vi "WaitForBytes.vi"(8 "error in (no error)":errorcluster, 10 "timeout [s]":i32, 11 "VISA Refnum in":refnum<visa-resource-name>) -> (0 "error out":errorcluster, 2 "Bytes at Port":u32, 3 "VISA Refnum out":refnum<visa-resource-name>)   [LabVIEW 2016]
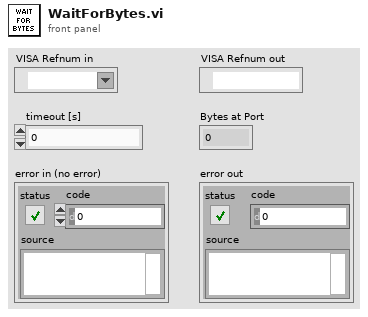
[diagram p1: front panel]
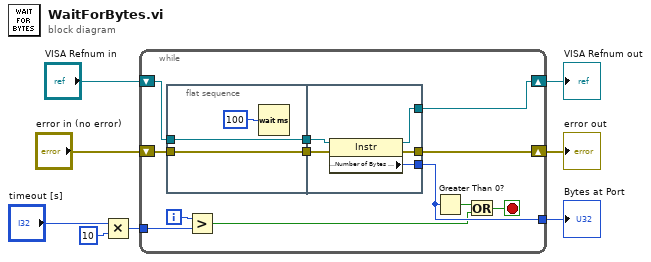
[diagram p0: block diagram]
diagram:
  n1 = Multiply(x="timeout [s]", y=10) -> (x*y=w8:i32)
  n2 = while {
    tunnel: [w16] -> w4
    shift-right: [w18] -> w3
    shift-left: "VISA Refnum in" -> [w20]
    shift-right: [w17] -> w5
    shift-left: "error in (no error)" -> [w19]
    tunnel: w8 -> [w9]
    i -> [w10]
    stop <- w12 stop-if-true
    n3 = flat-sequence {
      tunnel: w19 -> [w22]
      tunnel: w20 -> [w23]
      tunnel: [w23] -> w15
      tunnel: [w22] -> w14
      tunnel: [w26] -> w18
      tunnel: [w25] -> w17
      tunnel: [w24] -> w16
      tunnel: w15 -> [w28]
      tunnel: w14 -> [w27]
      frame #0 {
        n4 = Wait (ms)(milliseconds to wait=u32 100) -> ()  [unwired: 1 out]
      }
      frame #1 {
        n5 = property class="Instr"(reference=w28, error in=w27) -> (reference out=w26:refnum<visa-resource-name>, error out=w25:errorcluster, "Serial Settings:Number of Bytes at Serial Port"=w24:u32)
      }
    }
    n6 = Greater?(x=w10, y=w9) -> (0:w11:bool)
    n7 = Greater Than 0?(x=w16) -> (x > 0?=w13:bool)
    n8 = Or(x=w13, y=w11) -> (x .or. y?=w12:bool)
  }
  "error out" <- w5
  "Bytes at Port" <- w4
  "VISA Refnum out" <- w3
